vi "TurningPID.vi"(3 "PID gains":T1={"proportional gain (Kc)"=1.0, "integral time (Ti, min)"=0.01, "derivative time (Td, min)"=0.0} {"derivative time (Td, min)" format="%.3f"; "integral time (Ti, min)" format="%.3f"; "proportional gain (Kc)" format="%.3f"}, 4 "Invert Steering":bool, 5 "Tgt Angle":dbl format="%.2f", 6 "Current Angle":dbl format="%.2f") -> (0 "Right Motor %":dbl format="%.2f", 1 "Left Motor %":dbl format="%.2f", 2 "Angle Diff":dbl format="%.2f")   [LabVIEW 2015]
uses:
  <vilib>/addons/control/pid/pid.llb/PID (DBL).vi
  <vilib>/addons/control/pid/NI_PID_pid.lvlib
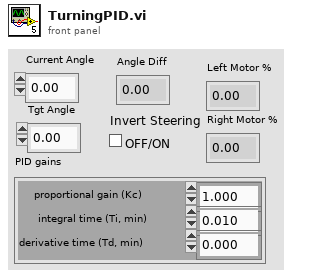
[diagram p1: front panel]
types:
  T1 = cluster{"proportional gain (Kc)":dbl, "integral time (Ti, min)":dbl, "derivative time (Td, min)":dbl}
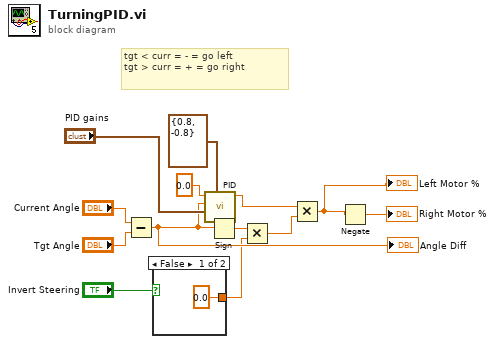
[diagram p0: block diagram]
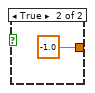
[diagram p2: hidden frame]
diagram:
  # "tgt < curr = - = go left\ntgt > curr = + = go right"
  n1 = Subtract(x="Current Angle", y="Tgt Angle") -> (x-y=w7:dbl)
  "Angle Diff" <- w7
  n2 = case shown="False" "Invert Steering" {
    tunnel: [0.0 -1.0] -> w2
    frame False {
    }
    frame True {
    }
  }
  n3 = call-poly <vilib>:"PID.vi"("output range"=cluster{"output high":dbl, "output low":dbl} {"output high"=0.8, "output low"=-0.8}, "PID gains"="PID gains", "process variable"=w7, "setpoint"=0.0) -> ("output"=w11:dbl)  [unwired: 6 in, 1 out]
  n4 = Sign(1:w7) -> (0:w3:dbl)
  n5 = Multiply(x=w3, y=w2) -> (x*y=w1:dbl)
  n6 = Multiply(x=w11, y=w1) -> (x*y=w5:dbl)
  "Left Motor %" <- w5
  n7 = Negate(x=w5) -> (-x=→"Right Motor %":dbl)
